vi "get_sjbumen_sp_gonghao.vi"(3 "juese":string, 6 "gonghao":string) -> (0 "error":errorcluster caption="error out 10", 1 "sp":string[][](array[string]))   [LabVIEW 2017, in "Lib_code.lvlib"]
uses:
  Lib_code.lvlib
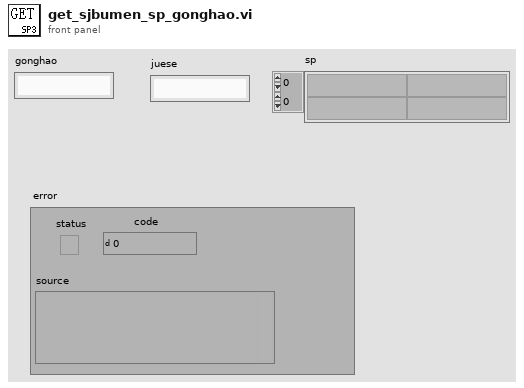
[diagram p1: front panel]
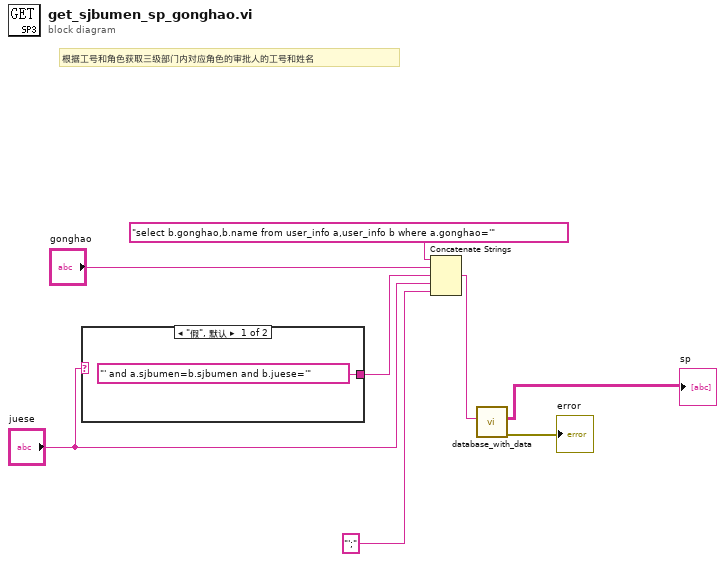
[diagram p0: block diagram]
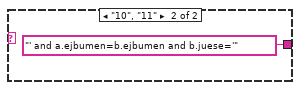
[diagram p2: hidden frame]
diagram:
  # "根据工号和角色获取三级部门内对应角色的审批人的工号和姓名"
  n1 = case shown="\"假\", 默认" "juese" {
    tunnel: ["' and a.sjbumen=b.sjbumen and b.juese='" ("字符串") "' and a.ejbumen=b.ejbumen and b.juese='" ("字符串")] -> w7
    frame "假", Default {
    }
    frame "10", "11" {
    }
  }
  n2 = Concatenate Strings("select b.gonghao,b.name from user_info a,user_info b where a.gonghao='" ("Command Text"), "gonghao", w7, "juese", "';" ("字符串")) -> (w4:string)
  n3 = call "database_with_data.vi"("input"=w4) -> ("error"=→"error":errorcluster, "Data"=→"sp":string[][])  [unwired: 9 in]
